vi "niDDC Abort.vi"(8 "error in (no error)":errorcluster, 11 "Class in":refnum<class "7976R_v1.lvclass">) -> (0 "error out":errorcluster, 3 "Class out":refnum<class "7976R_v1.lvclass">)   [LabVIEW 2015, in "7976R_v1.lvclass"]
uses:
  <userlib>/SE-APP-Receiver/NI5772/7976R_v1/7976R_v1.lvclass
  <userlib>/SE-APP-Receiver/NI5772/7976R_v1/7976R_v1.lvclass/7976R_v1.ctl
  <vilib>/Utility/error.llb/Error Cluster From Error Code.vi
  <vilib>/rvi/errors/niLvFpgaAdjustHostInterfaceError.vi
  <vilib>/rvi/interface/nirviReadWriteControl/nirviReadWriteControl.xnode
  <userlib>/SE-APP-Receiver/NI5772/7976R_v1/Private/FPGA VI Reference_DDC_v1.8.ctl
  NiFpgaLv.dll
  <vilib>/rvi/interface/Simulation/niFpgaSimulationCallBeginRW.vi
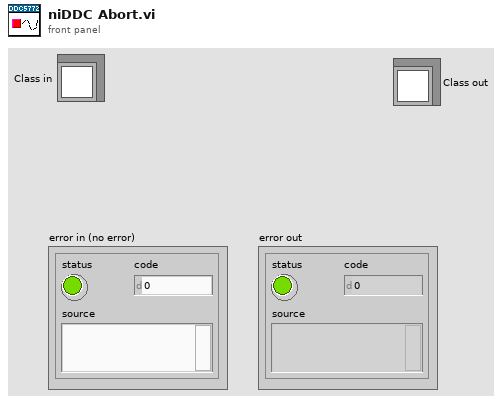
[diagram p1: front panel]
types:
  T1 = typedef "7976R_v1.lvclass/FPGA VI Reference_DDC_v1.8.ctl" = refnum<k20>
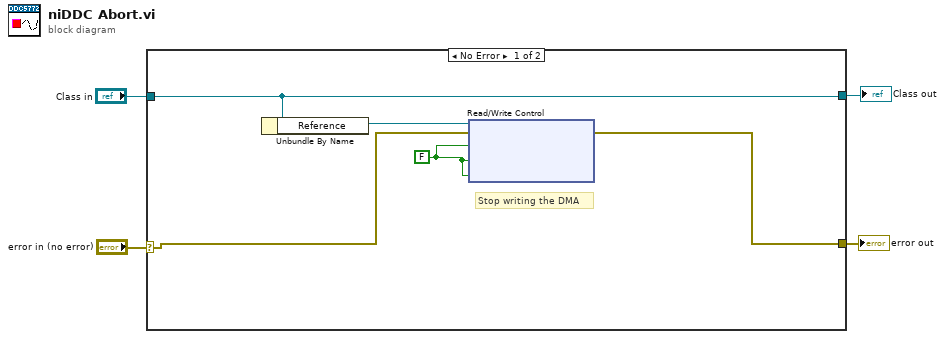
[diagram p0: block diagram]
diagram:
  n1 = case shown="No Error" "error in (no error)" {
    selector: "error in (no error)" -> [w7 w11]
    tunnel: [w6 w11] -> w4
    tunnel: "Class in" -> [w9 w10]
    tunnel: [w9 w10] -> w1
    frame No Error {
      w5 = FALSE
      # "Stop writing the DMA"
      n2 = Unbundle By Name(w9) -> ("Reference"=w8:T1)
      n3 = xnode "Read/Write Control"("FPGA VI Reference In"=w8, "error in"=w7, "dbg.stream.enable.2"=w5, "dbg.stream.enable.1"=w5, "mode.continuous"=w5) -> ("error out"=w6:errorcluster)  [unwired: 1 out]
    }
    frame Error {
    }
  }
  "error out" <- w4
  "Class out" <- w1
